vi "DB Select.vi"(6 "Select":enum16{"SelectWithQuery", "SelectWithColumn"}(ring)=enum."SelectWithColumn", 8 "error in (no error)":errorcluster, 9 "SQLTableData":T1, 10 "SQL query":string, 11 "Database in":refnum<class "Database.lvclass">) -> (0 "error out":errorcluster, 2 "data":string[][](array[string]), 3 "Database out":refnum<class "Database.lvclass">)   [LabVIEW 2023, in "HardwareAbstractionLayer_LVOOP.lvlib" / "Database.lvclass"]
uses:
  Database.lvclass
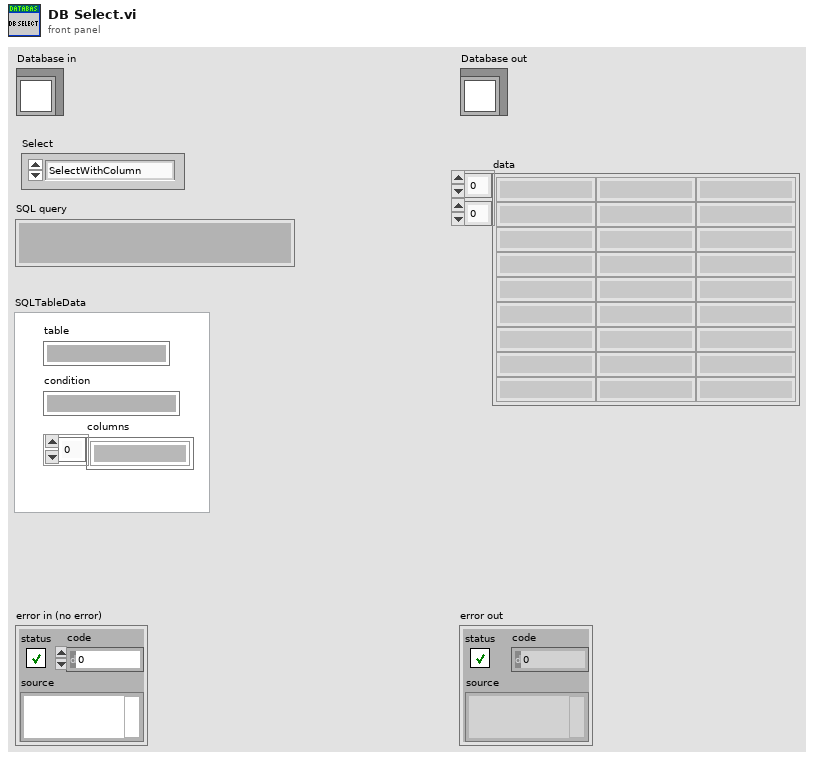
[diagram p1: front panel]
types:
  T1 = cluster{"table":string, "condition":string, "columns":string[]}
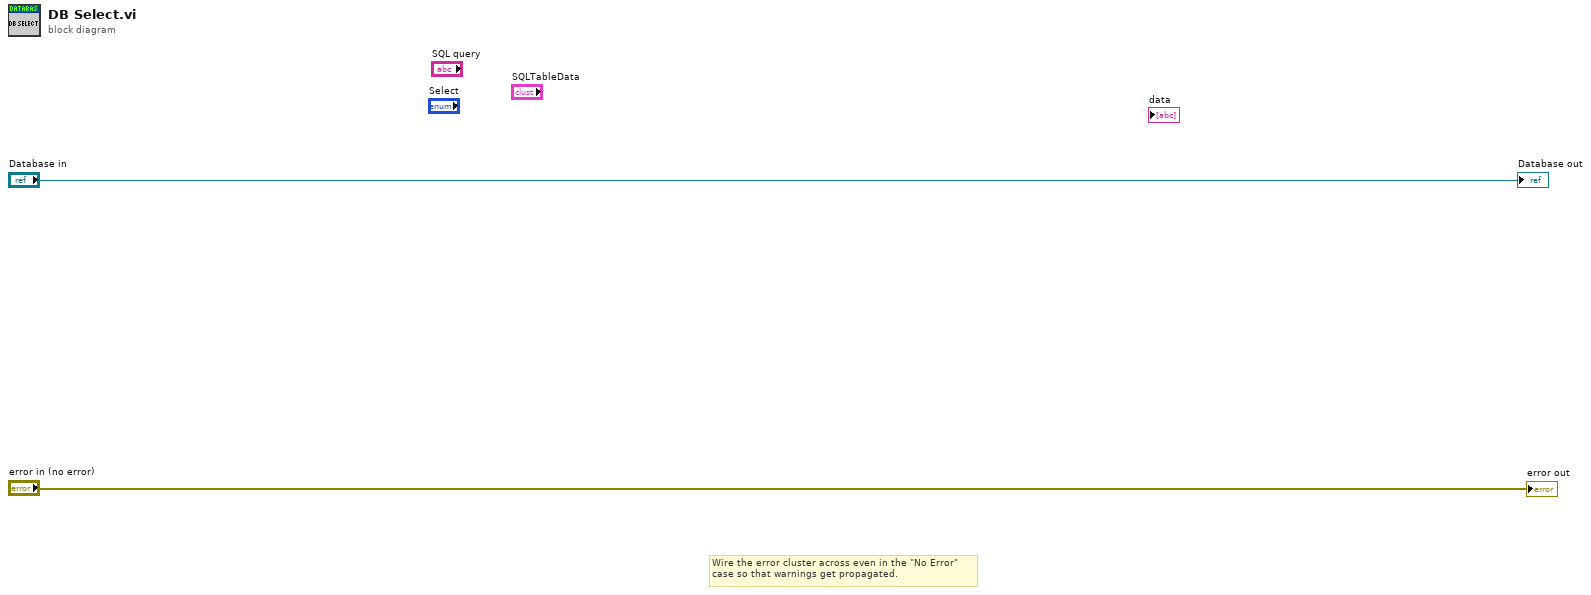
[diagram p0: block diagram]
diagram:
  # "Wire the error cluster across even in the \"No Error\"\ncase so that warnings get propagated."
  "error out" <- "error in (no error)"
  "Database out" <- "Database in"
